vi "error response to actions.vi"(11 "error handling":T2) -> (3 "actions":T1[](array[typedef]))   [LabVIEW 2013, in "Standard Engine Runtime.lvclass"]
uses:
  Standard Engine Runtime.lvclass
  Configuration/error options.ctl
  Configuration/Error Actions.ctl
  Configuration/Standard Engine Configuration.lvclass
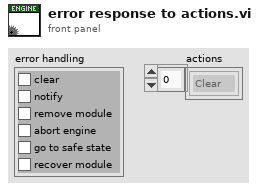
[diagram p1: front panel]
types:
  T1 = typedef "Standard Engine Configuration.lvclass/Error Actions.ctl" = enum16{"Clear", "Notify", "Stop Component", "Stop Engine", "Safe State", "Attempt Recovery"}
  T2 = typedef "Standard Engine Configuration.lvclass/error options.ctl" = cluster{"clear":bool, "notify":bool, "remove module":bool, "abort engine":bool, "go to safe state":bool, "recover module":bool}
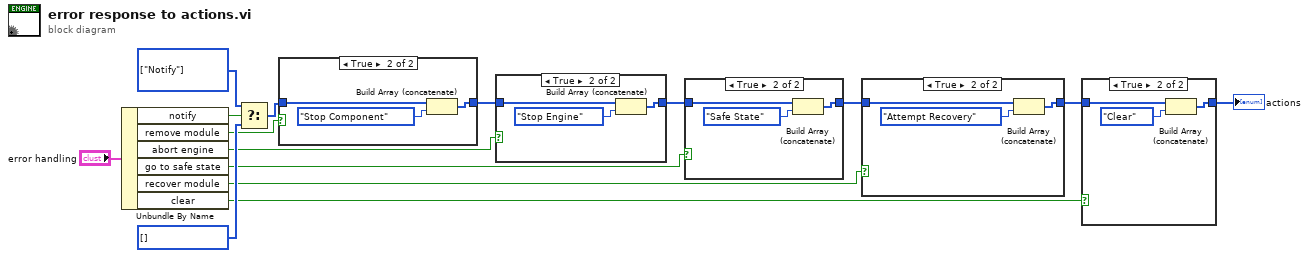
[diagram p0: block diagram]
diagram:
  w13 = T1[] [] items=["Clear", "Notify", "Stop Component", "Stop Engine", "Safe State", "Attempt Recovery"] ("actions")
  w12 = T1[] [enum."Notify"] items=["Clear", "Notify", "Stop Component", "Stop Engine", "Safe State", "Attempt Recovery"] ("actions")
  n1 = Unbundle By Name("error handling") -> ("notify"=w14:bool, "remove module"=w10:bool, "abort engine"=w6:bool, "go to safe state"=w5:bool, "recover module"=w4:bool, "clear"=w2:bool)
  n2 = Select(t=w12, s=w14, f=w13) -> (s? t:f=w11:T1[])
  n3 = case shown="True" w10 {
    tunnel: w11 -> [w16 w19]
    tunnel: [w16 w17] -> w9
    frame False {
    }
    frame True {
      n4 = Build Array (concatenate)(w19, Error_Actions."Stop Component" ("Error Actions")) -> (w17:T1[])
    }
  }
  n5 = case shown="True" w6 {
    tunnel: w9 -> [w20 w23]
    tunnel: [w20 w21] -> w8
    frame False {
    }
    frame True {
      n6 = Build Array (concatenate)(w23, Error_Actions."Stop Engine" ("Error Actions")) -> (w21:T1[])
    }
  }
  n7 = case shown="True" w5 {
    tunnel: w8 -> [w24 w27]
    tunnel: [w24 w25] -> w7
    frame False {
    }
    frame True {
      n8 = Build Array (concatenate)(w27, Error_Actions."Safe State" ("Error Actions")) -> (w25:T1[])
    }
  }
  n9 = case shown="True" w4 {
    tunnel: w7 -> [w28 w31]
    tunnel: [w28 w29] -> w3
    frame False {
    }
    frame True {
      n10 = Build Array (concatenate)(w31, Error_Actions."Attempt Recovery" ("Error Actions")) -> (w29:T1[])
    }
  }
  n11 = case shown="True" w2 {
    tunnel: w3 -> [w32 w35]
    tunnel: [w32 w33] -> w1
    frame False {
    }
    frame True {
      n12 = Build Array (concatenate)(w35, Error_Actions."Clear" ("Error Actions")) -> (w33:T1[])
    }
  }
  "actions" <- w1
